vi "SaveSizeDistributionfile.vi"(8 "error in (no error)":errorcluster, 10 "File path for Size dist analysis":path=path "\\\\psf\\Home/Desktop/Naama/FreezinProfile900C-26_12_2014-14_51_33.avi" caption="Path", 11 "Droplet Sizes (microns)":dbl[](array[numeric])) -> (0 "error out":errorcluster, 3 "Droplet Sizes (microns) 2":dbl[](array[numeric]))   [LabVIEW 2015]
doc: "Use this template to build a VI to use as a subVI."
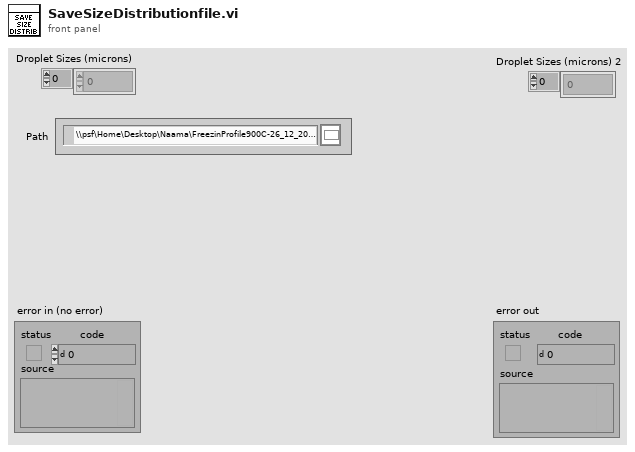
[diagram p1: front panel]
types:
  T1 = enum16{"open", "replace", "create", "open or create", "replace or create", "replace or create with confirmation"}
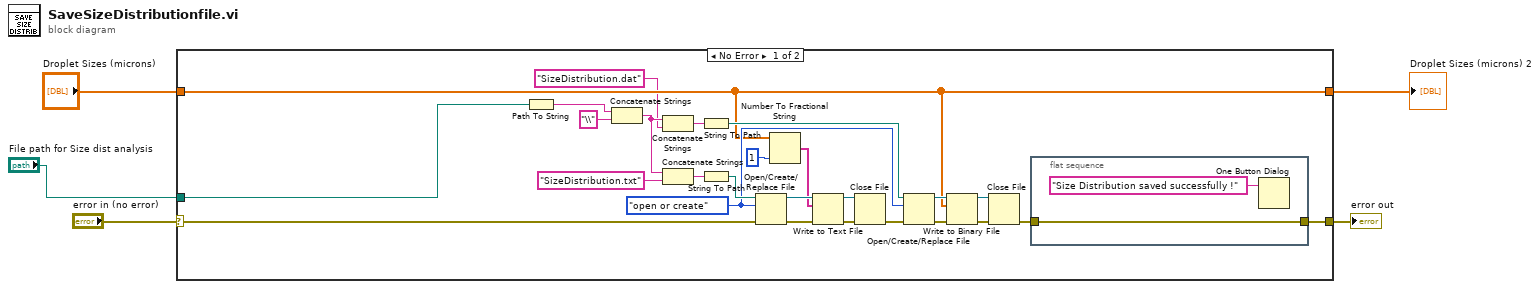
[diagram p0: block diagram]
diagram:
  n1 = case shown="No Error" "error in (no error)" {
    selector: "error in (no error)" -> [w6 w35]
    tunnel: [w26 w35] -> w4
    tunnel: "Droplet Sizes (microns)" -> [w14 w34]
    tunnel: [w14 w34] -> w2
    tunnel: "File path for Size dist analysis" -> [w7 _]
    frame No Error {
      w16 = T1."open or create" ("operation (0:open)")
      n2 = Path To String(path=w7) -> (string=w31:string)
      n3 = Concatenate Strings(w31, "\\" ("string")) -> (w9:string)
      n4 = Concatenate Strings(w9, "SizeDistribution.dat" ("string")) -> (w10:string)
      n5 = Concatenate Strings(w9, "SizeDistribution.txt" ("string")) -> (w11:string)
      n6 = String To Path(string=w10) -> (path=w15:path)
      n7 = String To Path(string=w11) -> (path=w27:path)
      n8 = Open/Create/Replace File(file path (use dialog)=w27, error in=w6, operation (0:open)=w16) -> (refnum out=w29:refnum<file>, error out=w28:errorcluster)  [unwired: 3 in, 1 out]
      n9 = Number To Fractional String(number=w14, precision (6)=i16 1) -> (F-format string=w23:string[])  [unwired: 2 in]
      n10 = Write to Text File(file (use dialog)=w29, text=w23, error in=w28) -> (refnum out=w25:refnum<file>, error out=w24:errorcluster)  [unwired: 1 in, 1 out]
      n11 = Close File(refnum=w25, error in=w24) -> (error out=w17:errorcluster)  [unwired: 1 out]
      n12 = Open/Create/Replace File(file path (use dialog)=w15, error in=w17, operation (0:open)=w16) -> (refnum out=w18:refnum<file>, error out=w19:errorcluster)  [unwired: 3 in, 1 out]
      n13 = Write to Binary File(file (use dialog)=w18, data=w14, error in=w19) -> (refnum out=w20:refnum<file>, error out=w21:errorcluster)  [unwired: 3 in, 1 out]
      n14 = Close File(refnum=w20, error in=w21) -> (error out=w13:errorcluster)  [unwired: 1 out]
      n15 = flat-sequence {
        tunnel: w13 -> [w33]
        tunnel: [w33] -> w26
        frame #0 {
          n16 = One Button Dialog(message="Size Distribution saved successfully !") -> ()  [unwired: 1 in, 1 out]
        }
      }
    }
    frame Error {
    }
  }
  "error out" <- w4
  "Droplet Sizes (microns) 2" <- w2
